vi "PCE PC Host.vi"() -> ()   [LabVIEW 2015]
uses:
  <vilib>/Utility/error.llb/Error Cluster From Error Code.vi
  <vilib>/rvi/errors/niLvFpgaAdjustHostInterfaceError.vi
  Globals.vi
  <vilib>/FPGAPlugInAG/Dynamic/niLvFpga_Close_Dynamic.vi
  <vilib>/rvi/interface/nirviMethod/nirviMethod.xnode
  <vilib>/rvi/interface/nirviCloseFPGA/nirviCloseFPGA.xnode
  <vilib>/rvi/interface/nirviReadWriteControl/nirviReadWriteControl.xnode
  <vilib>/rvi/interface/Simulation/niFpgaSimulationCallBeginRW.vi
  <vilib>/rvi/interface/nirviOpenFPGA/nirviOpenFPGA.xnode
  <vilib>/FPGAPlugInAG/Dynamic/niLvFpga_Reset_Dynamic.vi
  <vilib>/FPGAPlugInAG/Dynamic/niLvFpga_Run_Dynamic.vi
  Write Waveform to FPGA Folder/Write Waveform to FPGA.vi
  <vilib>/rvi/errors/niLvFpgaMergeErrorWithErrorCode.vi
  <vilib>/FPGAPlugInAG/Dynamic/niLvFpga_ReadFifo_Dynamic.vi
  NiFpgaLv.dll
  <vilib>/rvi/interface/RandomDataEmulation/nirviRandomDataOpen.vi
  <vilib>/rvi/interface/common/niFpgaCacheSessionInfoDynamic.vi
  <vilib>/FPGAPlugInAG/Dynamic/niLvFpga_WriteFifo_Dynamic.vi
panel:
  out "Request Done":bool
  out "Read Done":bool
  out "Write Done":bool
  out "Current Process":enum16{"Wait", "Write", "Read", "Stop"}(ring)
  out "Size of XY":i32
  out "WaveXY":u16[](graph)
  in  "Read Waveform":bool caption="元素入队列"
  in  "Resolution":u16(ring)=512 items=["2048*2048"=2048, "1024*1024"=1024, "512*512"=512, "256*256"=256]
  out "WaveX":u16[](graph)
  out "WaveY":u16[](graph)
  out "WaveXY":u16[](array[numeric])
  out "数组":u16[][](array[numeric])
  out "大小":i32[](array[numeric])
  out "Waveform to FIFO done":bool
  out "Events with Data":i32
  in  "stop":bool caption="停止"
  in  "Start Scanning":bool caption="元素入队列"
  in  "Load Waveform":bool caption="元素入队列"
  out "Galvo Waveform data X":path=path "C:/Users/hppc/Desktop/OpenScan/New Structure/waveX.txt"
  out "Waveform Points":i32=5120
  out "Galvo Waveform data Y":path=path "C:/Users/hppc/Desktop/OpenScan/New Structure/waveY.txt"
  in  "Initialize":bool caption="停止"
  out "error out":errorcluster
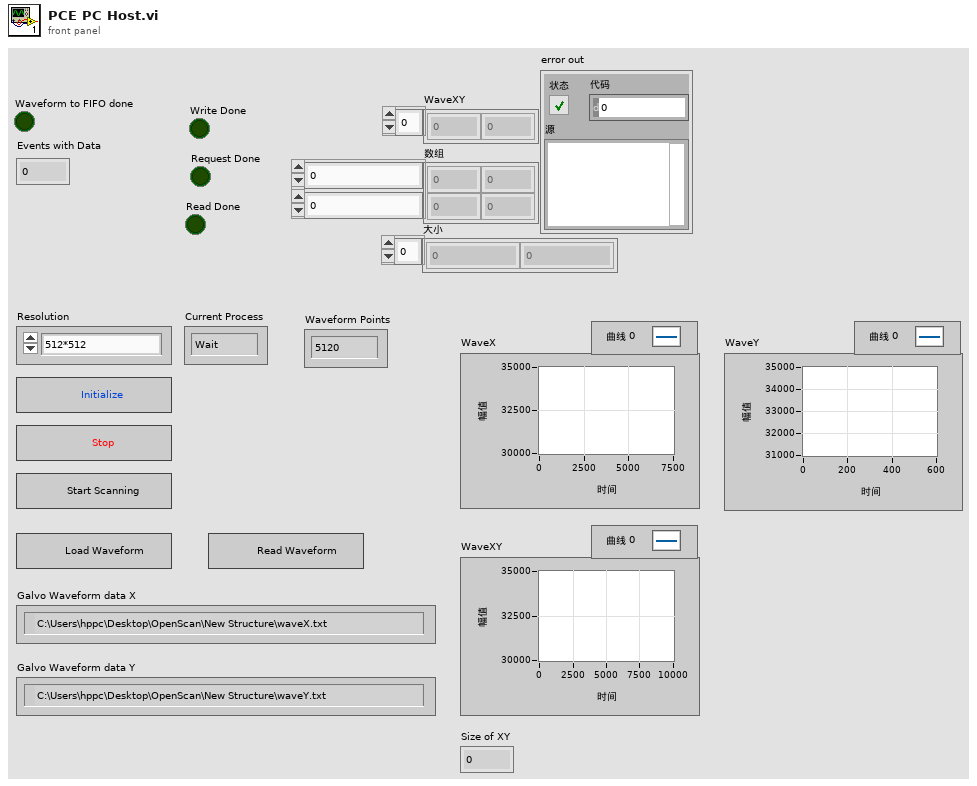
[diagram p1: front panel]
types:
  T1 = cluster{"FPGA VI引用输出":refnum<k20>, "错误输出":errorcluster}
  T2 = enum16{"Load Waveform", "Start Scanning", "Save Image", "Stop"}
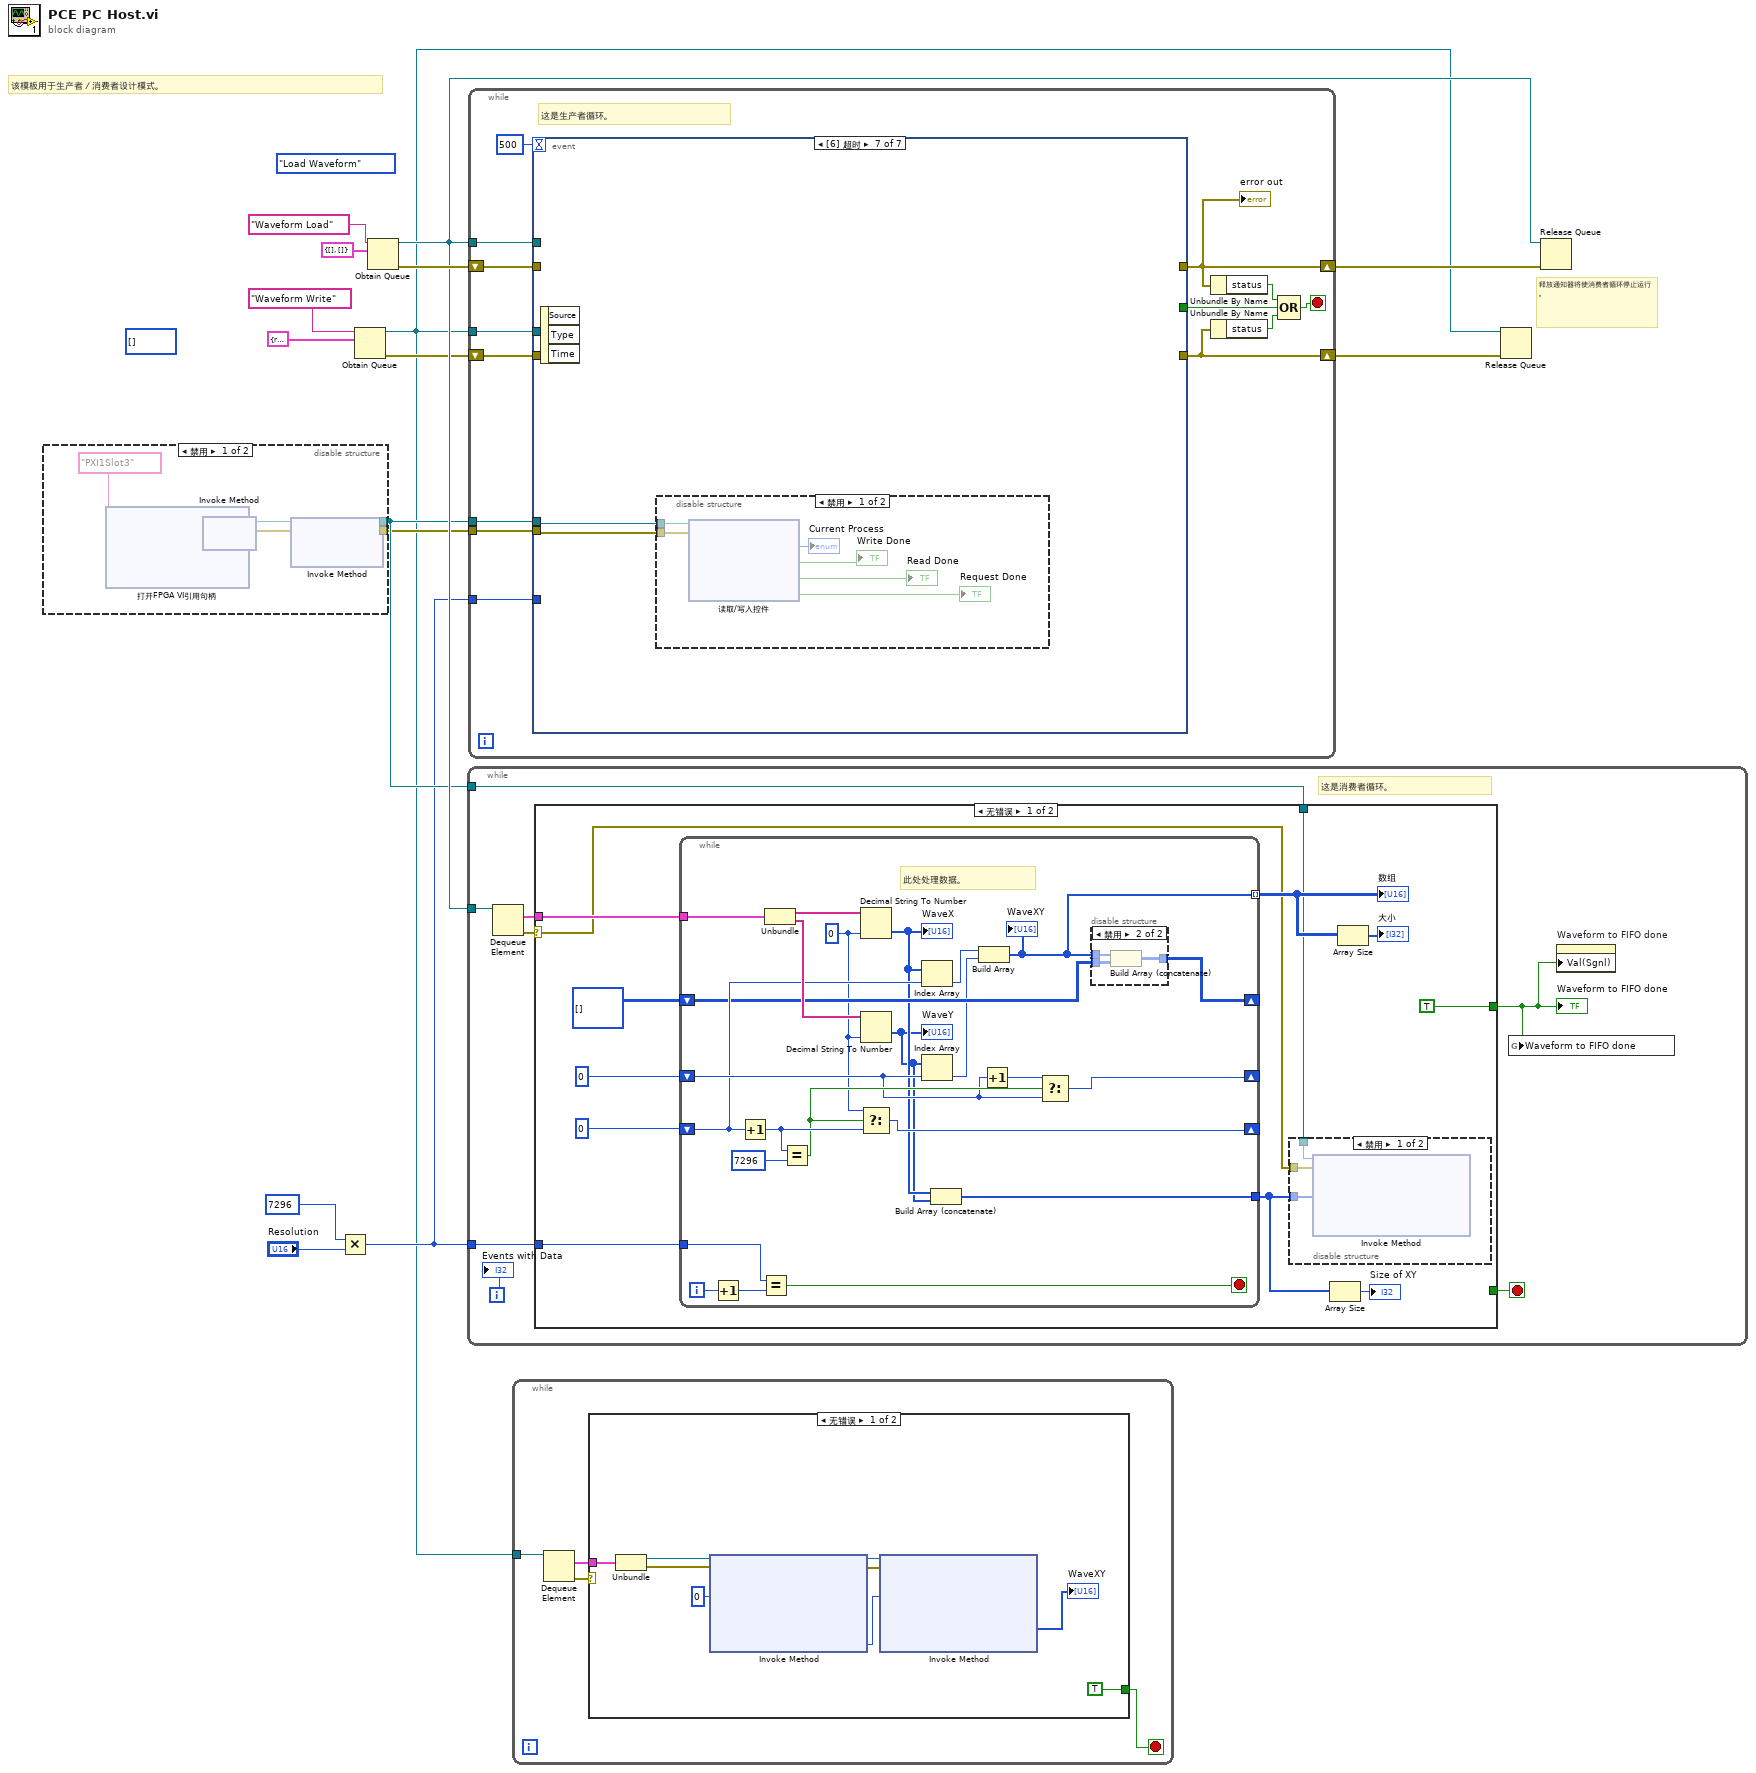
[diagram p0: block diagram]
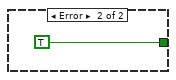
[diagram p2: hidden frame]
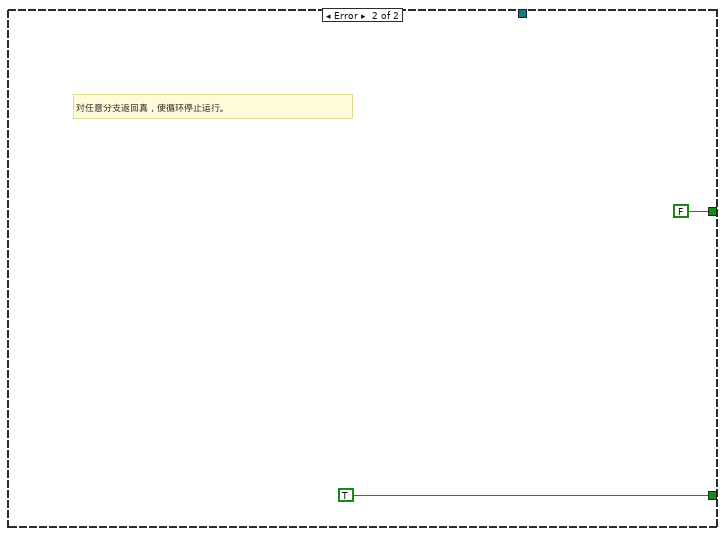
[diagram p6: hidden frame]
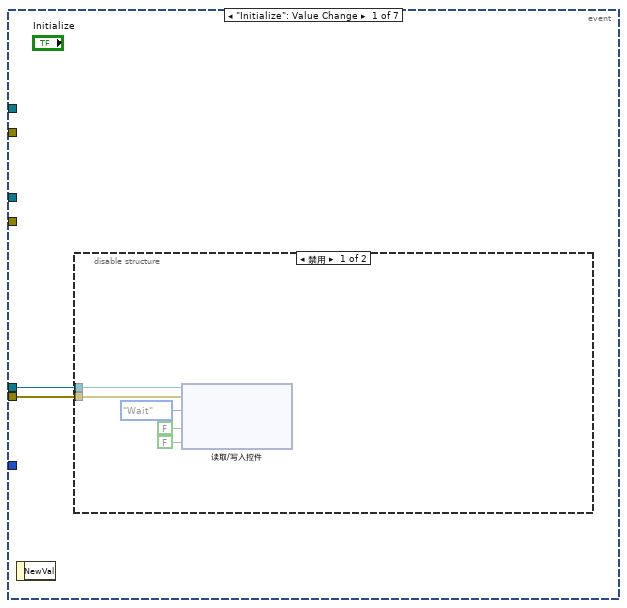
[diagram p7: hidden frame]
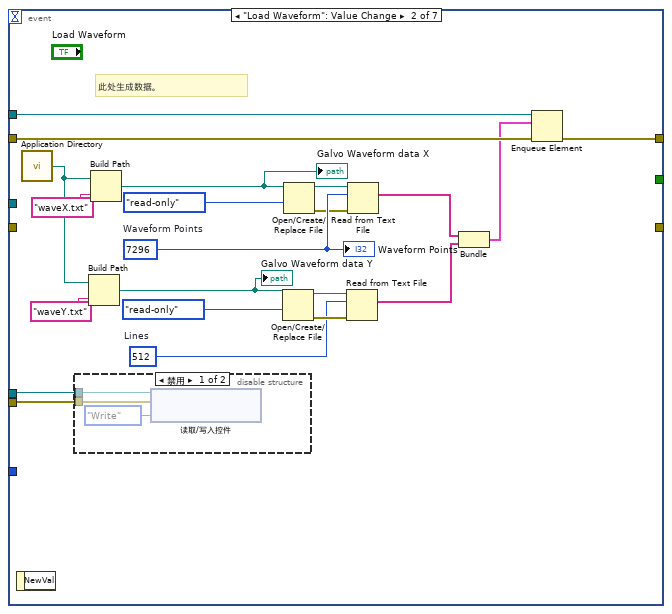
[diagram p9: hidden frame]
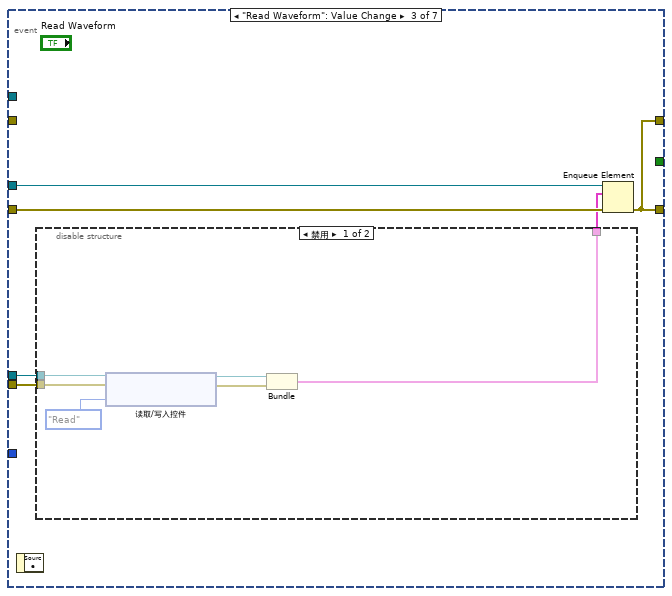
[diagram p11: hidden frame]
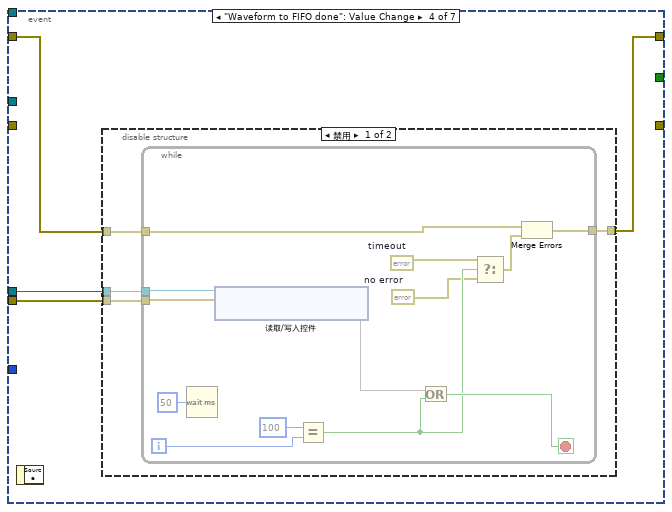
[diagram p13: hidden frame]
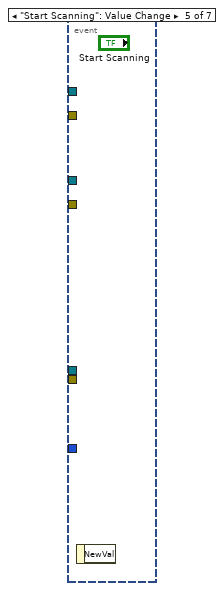
[diagram p15: hidden frame]
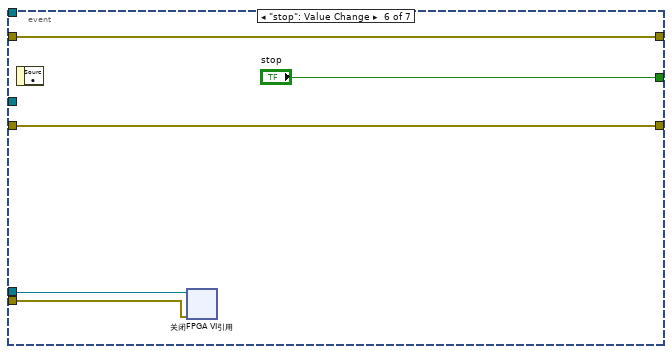
[diagram p16: hidden frame]
diagram:
  (unwired) u16[] [] ("数据")
  (unwired) T2."Load Waveform"
  # "释放通知器将使消费者循环停止运行。"
  # "该模板用于生产者／消费者设计模式。"
  n1 = disable-structure shown="禁用" {
    disable-tunnel: [w17 _] -> w11
    disable-tunnel: [w16 _] -> w10
    frame Disabled {
      n2 = xnode "打开FPGA VI引用句柄"("资源名称"=tag "PXI1Slot3") -> ("FPGA VI引用输出"=w21:refnum<k20>, "错误输出"=w20:errorcluster)  [unwired: 1 in]
      n3 = xnode "Invoke Method"("FPGA VI引用输入"=w21, "错误输入"=w20) -> ("FPGA VI引用输出"=w19:refnum<k20>, "错误输出"=w18:errorcluster)
      n4 = xnode "Invoke Method"("FPGA VI引用输入"=w19, "错误输入"=w18) -> ("FPGA VI引用输出"=w17:refnum<k20>, "错误输出"=w16:errorcluster)  [unwired: 1 in]
    }
    frame Enabled {
    }
  }
  n5 = Multiply(x=7296, y="Resolution") -> (x*y=w7:i32)
  n6 = Obtain Queue(name (unnamed)="Waveform Write" ("名称（未命名）"), element data type=T1 {"FPGA VI引用输出"=refnum, "错误输出"={"status"=FALSE, "code"=0, "source"=""}} ("输出簇")) -> (queue out=w3:refnum<queue>, error out=w4:errorcluster)  [unwired: 3 in, 1 out]
  n7 = Obtain Queue(name (unnamed)="Waveform Load" ("名称（未命名）"), element data type=cluster{string[], string[]} {[], []} ("输出簇")) -> (queue out=w13:refnum<queue>, error out=w15:errorcluster)  [unwired: 3 in, 1 out]
  n8 = while {
    tunnel: w13 -> [w30]
    tunnel: w7 -> [w26]
    tunnel: w11 -> [w25]
    i -> [w24]
    stop <- w28 stop-if-true
    # "这是消费者循环。"
    n9 = Dequeue Element(queue=w30) -> (element=w27:cluster{string[], string[]}, error out=w29:errorcluster)  [unwired: 2 in, 2 out]
    n10 = case shown="无错误" w29 {
      selector: w29 -> [w34 _]
      tunnel: [_ TRUE] -> w28
      tunnel: w27 -> [w42 _]
      tunnel: w26 -> [w38 _]
      tunnel: w25 -> [w35 _]
      tunnel: [TRUE FALSE] -> w23
      frame No Error {
        n11 = while {
          tunnel: w42 -> [w69]
          shift-right: [w61] -> _
          shift-left: 0 ("索引") -> [w62]
          shift-right: [w65] -> _
          shift-left: 0 ("索引") -> [w60]
          shift-right: [w54] -> _
          shift-left: u16[][] [] ("添加的数组") -> [w59]
          tunnel: w38 -> [w56]
          tunnel: [w52] -> w36 mode=indexing
          tunnel: [w46] -> w32
          i -> [w57]
          stop <- w58 stop-if-true
          w53 = u16 0 ("默认(0 I32)")
          # "此处处理数据。"
          n12 = Increment(x=w57) -> (x+1=w55:i32)
          n13 = Increment(x=w60) -> (x+1=w66:i32)
          n14 = Equal?(x=w56, y=w55) -> (x = y?=w58:bool)
          n15 = Unbundle(w69) -> (w49:string[], w68:string[])
          n16 = Equal?(x=w66, y=7296) -> (x = y?=w64:bool)
          n17 = Decimal String To Number(string=w49, default (0L)=w53) -> (number=w48:u16[])  [unwired: 1 in, 1 out]
          "WaveX" <- w48
          n18 = Decimal String To Number(string=w68, default (0L)=w53) -> (number=w47:u16[])  [unwired: 1 in, 1 out]
          "WaveY" <- w47
          n19 = Select(t=w53, s=w64, f=w66) -> (s? t:f=w65:i32)
          n20 = Index Array(array=w48, index=w60) -> (element=w51:u16)
          n21 = Index Array(array=w47, index=w62) -> (element=w50:u16)
          n22 = Build Array (concatenate)(w48, w47) -> (w46:u16[])
          n23 = Build Array(w51, w50) -> (w52:u16[])
          "WaveXY" <- w52
          n24 = Increment(x=w62) -> (x+1=w63:i32)
          n25 = Select(t=w63, s=w64, f=w62) -> (s? t:f=w61:i32)
          n26 = disable-structure shown="禁用" {
            disable-tunnel: w59 -> [_ w72]
            disable-tunnel: [_ w71] -> w54
            disable-tunnel: w52 -> [_ w70]
            frame Enabled {
            }
            frame Disabled {
              n27 = Build Array (concatenate)(w70, w72) -> (w71:u16[][])
            }
          }
        }
        "数组" <- w36
        n28 = disable-structure shown="禁用" {
          disable-tunnel: w35 -> [w45 _]
          disable-tunnel: w34 -> [w44 _]
          disable-tunnel: w32 -> [w43 _]
          frame Disabled {
            n29 = xnode "Invoke Method"("FPGA VI引用输入"=w45, "错误输入"=w44, "数据"=w43) -> ()  [unwired: 1 in, 3 out]
          }
          frame Enabled {
          }
        }
        n30 = Array Size(array=w32) -> (size(s)=→"Size of XY":i32)
        n31 = Array Size(array=w36) -> (size(s)=→"大小":i32[])
      }
      frame Error {
        # "对任意分支返回真，使循环停止运行。"
      }
    }
    "Waveform to FIFO done" <- w23
    n32 = global write "Globals.vi" "Waveform to FIFO done"(w23) -> ()
    n33 = property on="Waveform to FIFO done" class="Bool (严格)"("Val(Sgnl)"=w23) -> ()  [unwired: 2 in, 2 out]
    "Events with Data" <- w24
  }
  n34 = while {
    shift-right: [w84] -> w14
    shift-left: w15 -> [w87]
    tunnel: w13 -> [w88]
    tunnel: w10 -> [w81]
    tunnel: w7 -> [w80]
    tunnel: w11 -> [w82]
    tunnel: w3 -> [w79]
    shift-right: [w75] -> w2
    shift-left: w4 -> [w78]
    stop <- w85 stop-if-true
    # "这是生产者循环。"
    n35 = event shown="[6] 超时" {
      selector: _ -> [_ _ _ _ _ _ _]
      dyn-events: _ -> [_ _ _ _ _ _ _]
      timeout: 500 -> [_ _ _ _ _ _ _]
      tunnel: w88 -> [_ w116 _ _ _ _ _]
      tunnel: w87 -> [_ w115 _ w132 _ w156 _]
      tunnel: [_ w114 w121 w133 _ w156 _] -> w84
      tunnel: [_ _ _ _ _ "stop" _] -> w86
      tunnel: w82 -> [w90 w102 w125 w135 _ w154 w159]
      tunnel: w81 -> [w89 w101 w124 w134 _ w153 w158]
      tunnel: w80 -> [_ _ _ _ _ _ _]
      tunnel: w79 -> [_ _ w123 _ _ _ _]
      tunnel: w78 -> [_ _ w122 _ _ w155 _]
      tunnel: [_ _ w121 _ _ w155 _] -> w75
      event "Initialize": Value Change {
        n36 = event-data() -> ()  [unwired: 1 in, 1 out]
        n37 = disable-structure shown="禁用" {
          disable-tunnel: w90 -> [w95 _]
          disable-tunnel: w89 -> [w94 _]
          frame Disabled {
            n38 = xnode "读取/写入控件"("FPGA VI引用输入"=w95, "错误输入"=w94, "Current Process"=enum16{"Wait", "Write", "Read", "Stop"}."Wait", "Write Done"=FALSE, "Read Done"=FALSE) -> ()  [unwired: 2 out]
          }
          frame Enabled {
          }
        }
      }
      event "Load Waveform": Value Change {
        w108 = 512  # Lines
        w111 = 7296  # Waveform Points
        # "此处生成数据。"
        n39 = event-data() -> ()  [unwired: 1 in, 1 out]
        n40 = call <vilib>:"Application Directory.vi"() -> ("Application Directory"=w98:path)
        n41 = disable-structure shown="禁用" {
          disable-tunnel: w102 -> [w119 _]
          disable-tunnel: w101 -> [w118 _]
          frame Disabled {
            n42 = xnode "读取/写入控件"("FPGA VI引用输入"=w119, "错误输入"=w118, "Current Process"=enum16{"Wait", "Write", "Read", "Stop"}."Write") -> ()  [unwired: 2 out]
          }
          frame Enabled {
          }
        }
        n43 = Build Path(base path=w98, name or relative path="waveY.txt" ("名称或相对路径")) -> (appended path=w96:path)
        "Galvo Waveform data Y" <- w96
        n44 = Build Path(base path=w98, name or relative path="waveX.txt" ("名称或相对路径")) -> (appended path=w97:path)
        "Galvo Waveform data X" <- w97
        n45 = Open/Create/Replace File(file path (use dialog)=w96, access (0:read/write)=enum16{"read/write", "read-only", "write-only"}."read-only" ("权限(0:read/write)")) -> (refnum out=w107:refnum<file>, error out=w109:errorcluster)  [unwired: 4 in, 1 out]
        n46 = Open/Create/Replace File(file path (use dialog)=w97, access (0:read/write)=enum16{"read/write", "read-only", "write-only"}."read-only" ("权限(0:read/write)")) -> (refnum out=w112:refnum<file>, error out=w110:errorcluster)  [unwired: 4 in, 1 out]
        n47 = Read from Text File(file (use dialog)=w107, count=w108, error in=w109) -> (text=w105:string[])  [unwired: 1 in, 3 out]
        n48 = Read from Text File(file (use dialog)=w112, count=w111, error in=w110) -> (text=w103:string[])  [unwired: 1 in, 3 out]
        n49 = Bundle(w103, w105) -> (w104:cluster{string[], string[]})  [unwired: 1 in]
        n50 = Enqueue Element(queue=w116, element=w104, error in (no error)=w115) -> (error out=w114:errorcluster)  [unwired: 1 in, 2 out]
        "Waveform Points" <- w111
      }
      event "Read Waveform": Value Change {
        n51 = event-data() -> ()  [unwired: 1 in, 1 out]
        n52 = disable-structure shown="禁用" {
          disable-tunnel: w125 -> [w130 _]
          disable-tunnel: w124 -> [w129 _]
          disable-tunnel: [w126 _] -> w120
          frame Disabled {
            n53 = xnode "读取/写入控件"("FPGA VI引用输入"=w130, "错误输入"=w129, "Current Process"=enum16{"Wait", "Write", "Read", "Stop"}."Read") -> ("FPGA VI引用输出"=w128:refnum<k20>, "错误输出"=w127:errorcluster)
            n54 = Bundle("FPGA VI引用输出"=w128, "错误输出"=w127) -> (w126:T1)  [unwired: 1 in]
          }
          frame Enabled {
          }
        }
        n55 = Enqueue Element(queue=w123, element=w120, error in (no error)=w122) -> (error out=w121:errorcluster)  [unwired: 1 in, 2 out]
      }
      event "Waveform to FIFO done": Value Change {
        n56 = event-data() -> ()  [unwired: 1 in, 1 out]
        n57 = disable-structure shown="禁用" {
          disable-tunnel: w135 -> [w139 _]
          disable-tunnel: w134 -> [w138 _]
          disable-tunnel: [w137 _] -> w133
          disable-tunnel: w132 -> [w136 _]
          frame Disabled {
            n58 = while {
              tunnel: w139 -> [w152]
              tunnel: w138 -> [w151]
              tunnel: [w145] -> w137
              tunnel: w136 -> [w144]
              i -> [w149]
              stop <- w146 stop-if-true
              w141 = errorcluster {"status"=FALSE, "code"=0, "source"=""}  # no error
              w142 = errorcluster {"status"=TRUE, "code"=0, "source"="Write Waveform DRAM timeout"}  # timeout
              n59 = Wait (ms)(milliseconds to wait=u32 50 ("等待时间（毫秒）")) -> ()  [unwired: 1 out]
              n60 = xnode "读取/写入控件"("FPGA VI引用输入"=w152, "错误输入"=w151) -> ("Waveform DRAM done"=w147)  [unwired: 2 out]
              n61 = Equal?(x=100, y=w149) -> (x = y?=w143:bool)
              n62 = Or(x=w147, y=w143) -> (x .or. y?=w146:bool)
              n63 = Select(t=w142, s=w143, f=w141) -> (s? t:f=w140:errorcluster)
              n64 = Merge Errors(w144, w140) -> (w145:errorcluster)
            }
          }
          frame Enabled {
          }
        }
      }
      event "Start Scanning": Value Change {
        n65 = event-data() -> ()  [unwired: 1 in, 1 out]
      }
      event "stop": Value Change {
        n66 = event-data() -> ()  [unwired: 1 in, 1 out]
        n67 = xnode "关闭FPGA VI引用"("FPGA VI引用输入"=w154, "错误输入"=w153) -> ()  [unwired: 1 out]
      }
      event Timeout {
        n68 = event-data() -> ()  [unwired: 1 in, 3 out]
        n69 = disable-structure shown="禁用" {
          disable-tunnel: w159 -> [w165 _]
          disable-tunnel: w158 -> [w164 _]
          frame Disabled {
            n70 = xnode "读取/写入控件"("FPGA VI引用输入"=w165, "错误输入"=w164) -> ("Current Process"=→"Current Process":enum16{"Wait", "Write", "Read", "Stop"}, "Write Done"=→"Write Done":bool, "Read Done"=→"Read Done":bool, "Request Done"=→"Request Done":bool)  [unwired: 2 out]
          }
          frame Enabled {
          }
        }
      }
    }
    "error out" <- w84
    n71 = Unbundle By Name(w84) -> ("status"=w83:bool)
    n72 = Unbundle By Name(w75) -> ("status"=w76:bool)
    n73 = Compound Arithmetic op=OR ("复合运算")(w83, w86, w76) -> (w85:bool)
  }
  n74 = while {
    tunnel: w3 -> [w168]
    stop <- w166 stop-if-true
    n75 = Dequeue Element(queue=w168) -> (element=w167:T1, error out=w169:errorcluster)  [unwired: 2 in, 2 out]
    n76 = case shown="无错误" w169 {
      tunnel: w167 -> [w174 _]
      tunnel: [TRUE TRUE] -> w166
      frame No Error {
        n77 = Unbundle(w174) -> ("FPGA VI引用输出"=w173:refnum<k20>, "错误输出"=w172:errorcluster)
        n78 = xnode "Invoke Method"("FPGA VI引用输入"=w173, "错误输入"=w172, "元素数量"=u32 0) -> ("FPGA VI引用输出"=w177:refnum<k20>, "错误输出"=w171:errorcluster, "剩余元素"=w175:u32)  [unwired: 1 in, 1 out]
        n79 = xnode "Invoke Method"("FPGA VI引用输入"=w177, "错误输入"=w171, "元素数量"=w175) -> ("数据"=→"WaveXY":u16[])  [unwired: 1 in, 3 out]
      }
      frame Error {
      }
    }
  }
  n80 = Release Queue(queue=w3, error in (no error)=w2) -> ()  [unwired: 1 in, 3 out]
  n81 = Release Queue(queue=w13, error in (no error)=w14) -> ()  [unwired: 1 in, 3 out]
